vi "ABR-Plot Waveforms.vi"(0 "Array":dbl[][](array[numeric]), 2 "graph ref":refnum<vi>, 5 "dt (us)":dbl, 7 "Normalize traces":bool, 9 "Seqvals":dbl[](array[numeric]), 11 "error in (no error)":errorcluster, 12 "InnerVals":dbl[](array[numeric]), 13 "Threshold":dbl=nan) -> (15 "error out":errorcluster)   [LabVIEW 2020]
uses:
  epl-vi-lib/Utility VIs/Math VIs/LinSpace (x0-dx-npts).vi
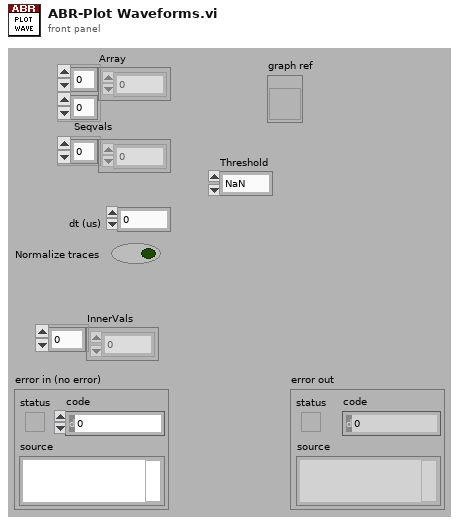
[diagram p1: front panel]
types:
  T1 = cluster{"Name":string, "Color":u32, "Style":u8, "Point Style":u8, "Name Visible":bool, "Allow Drag":bool, "Annotation Mode":u32, "Plot":i32, "Index":i32, "Position":cluster{"X":dbl, "Y":dbl}, "X Scale":u32, "Y Scale":u32, "Show Arrow":bool, "Lock Name":bool, "Plot Area":i32, "Label Offset":cluster{"X":dbl, "Y":dbl}}
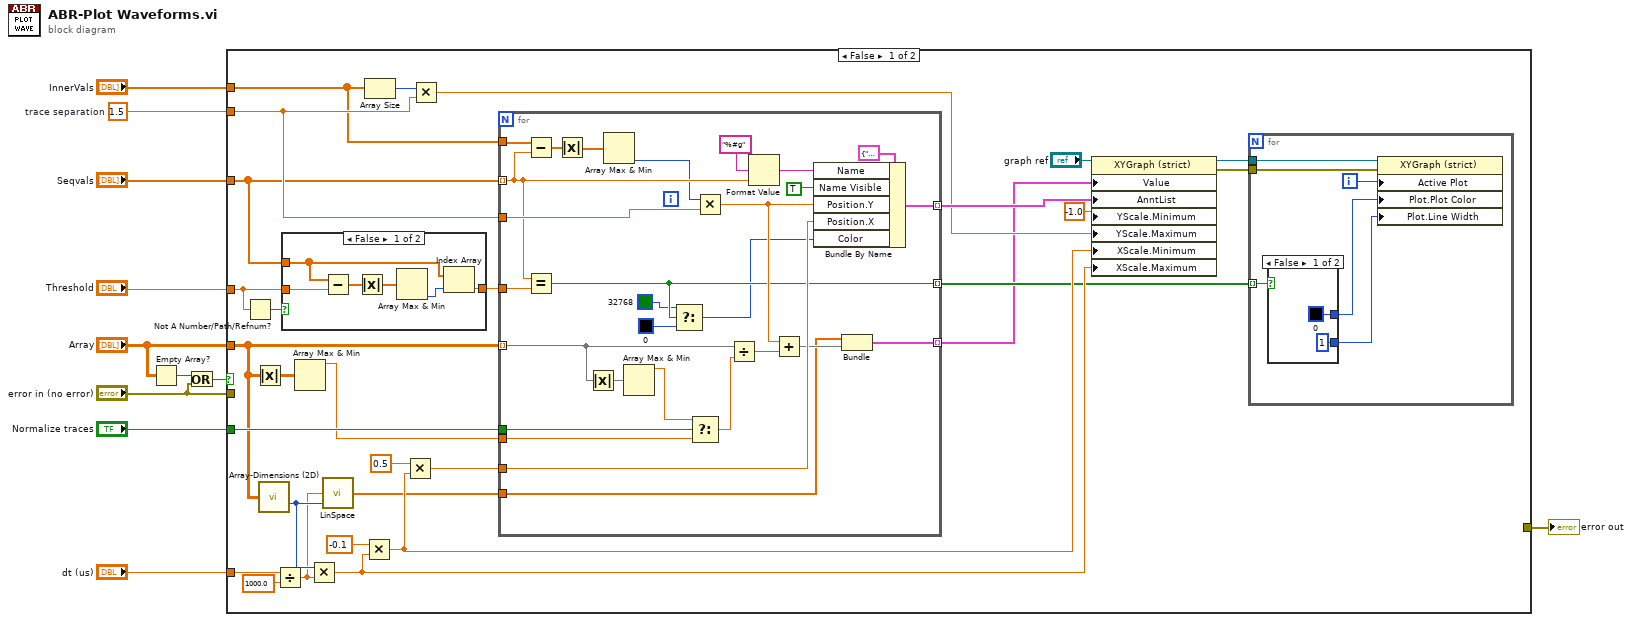
[diagram p0: block diagram]
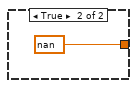
[diagram p2: hidden frame]
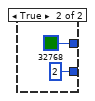
[diagram p3: hidden frame]
diagram:
  w8 = 1.5  # trace separation
  n1 = Empty Array?(array="Array") -> (empty?=w5:bool)
  n2 = Or(x=w5, y="error in (no error)") -> (x .or. y?=w3:bool)
  n3 = case shown="False" w3 {
    tunnel: "Array" -> [w30 _]
    tunnel: "dt (us)" -> [w40 _]
    tunnel: [_ w86] -> w10
    tunnel: "Seqvals" -> [w17 _]
    tunnel: w8 -> [w35 _]
    tunnel: "Normalize traces" -> [w33 _]
    tunnel: "InnerVals" -> [w24 _]
    tunnel: "error in (no error)" -> [_ w86]
    tunnel: "Threshold" -> [w14 _]
    frame False {
      n4 = Not A Number/Path/Refnum?(number/path/refnum=w14) -> (NaN/Path/Refnum?=w13:bool)
      n5 = Absolute Value(x=w30) -> (abs(x)=w32:dbl[][])
      n6 = call "Array-Dimensions (2D).vi"("2D Array"=w30) -> ("# columns"=w22:i32)  [unwired: 13 in, 1 out]
      n7 = Divide(x=w40, y=1000.0) -> (x/y=w20:dbl)
      n8 = case shown="False" w13 {
        tunnel: w17 -> [w43 _]
        tunnel: [w41 nan] -> w16
        tunnel: w14 -> [w44 _]
        frame False {
          n9 = Subtract(x=w43, y=w44) -> (x-y=w46:dbl[])
          n10 = Absolute Value(x=w46) -> (abs(x)=w45:dbl[])
          n11 = Array Max & Min(array=w45) -> (min index (indices)=w42:i32)  [unwired: 3 out]
          n12 = Index Array(array=w43, index=w42) -> (element=w41:dbl)
        }
        frame True {
        }
      }
      n13 = Array Max & Min(array=w32) -> (max value=w31:dbl)  [unwired: 3 out]
      n14 = Multiply(x=w22, y=w20) -> (x*y=w29:dbl)
      n15 = call-poly "LinSpace.vi"("npts"=w22, "dx"=w20) -> ("Array"=w21:dbl[])  [unwired: 2 in, 1 out]
      n16 = Multiply(x=-0.1, y=w29) -> (x*y=w26:dbl)
      n17 = Array Size(array=w24) -> (size(s)=w25:i32)
      n18 = Multiply(x=0.5, y=w26) -> (x*y=w23:dbl)
      n19 = Multiply(x=w25, y=w35) -> (x*y=w34:dbl)
      n20 = for {
        tunnel: w30 -> [w84] mode=indexing
        tunnel: [w69] -> w12 mode=indexing
        tunnel: w17 -> [w61] mode=indexing
        tunnel: [w80] -> w37 mode=indexing
        tunnel: w35 -> [w79]
        tunnel: w33 -> [w76]
        tunnel: w31 -> [w73]
        tunnel: w24 -> [w62]
        tunnel: w23 -> [w71]
        tunnel: w21 -> [w68]
        tunnel: w16 -> [w67]
        tunnel: [w66] -> w15 mode=indexing
        n21 = Subtract(x=w62, y=w61) -> (x-y=w60:dbl[])
        n22 = Equal?(x=w61, y=w67) -> (x = y?=w66:bool)
        n23 = Absolute Value(x=w60) -> (abs(x)=w59:dbl[])
        n24 = Absolute Value(x=w84) -> (abs(x)=w85:dbl[])
        n25 = Array Max & Min(array=w59) -> (min index (indices)=w58:i32)  [unwired: 3 out]
        n26 = Array Max & Min(array=w85) -> (max value=w75:dbl)  [unwired: 3 out]
        n27 = Select(t=u32 32768, s=w66, f=u32 0) -> (s? t:f=w63:u32)
        n28 = Select(t=w75, s=w76, f=w73) -> (s? t:f=w74:dbl)
        n29 = Multiply(x=w58, y=w79) -> (x*y=w78:dbl)
        n30 = Divide(x=w84, y=w74) -> (x/y=w77:dbl[])
        n31 = Format Value(format string="%#g", value (0)=w61) -> (output string=w81:string)  [unwired: 1 in]
        n32 = Add(x=w78, y=w77) -> (x+y=w70:dbl[])
        n33 = Bundle By Name(cluster=T1 {"Name"="", "Color"=0, "Style"=0, "Point Style"=0, "Name Visible"=FALSE, "Allow Drag"=FALSE, "Annotation Mode"=0, "Plot"=0, "Index"=0, "Position"={"X"=0.0, "Y"=0.0}, "X Scale"=0, "Y Scale"=0, "Show Arrow"=FALSE, "Lock Name"=FALSE, "Plot Area"=0, "Label Offset"={"X"=0.0, "Y"=0.0}} ("dummy annotation cluster\n(so we can bundle by name)"), "Name"=w81, "Name Visible"=TRUE, "Position.Y"=w78, "Position.X"=w71, "Color"=w63) -> (w80:T1)
        n34 = Bundle("Array"=w68, w70) -> (w69:cluster{"Array":dbl[], dbl[]})  [unwired: 1 in]
      }
      n35 = property class="XYGraph (strict)"(reference="graph ref", "Value"=w12, "AnntList"=w37, "YScale.Minimum"=-1.0 ("Y Scale.Range:Minimum"), "YScale.Maximum"=w34, "XScale.Minimum"=w26, "XScale.Maximum"=w29) -> (reference out=w19:refnum<vi>, error out=w18:errorcluster)  [unwired: 1 in]
      n36 = for {
        tunnel: w19 -> [w53]
        tunnel: w18 -> [w52]
        tunnel: w15 -> [w48] mode=indexing
        i -> [w51]
        n37 = case shown="False" w48 {
          tunnel: [u32 0 u32 32768] -> w50
          tunnel: [1 2] -> w49
          frame False {
          }
          frame True {
          }
        }
        n38 = property class="XYGraph (strict)"(reference=w53, error in=w52, "Active Plot"=w51, "Plot.Plot Color"=w50, "Plot.Line Width"=w49) -> ()  [unwired: 2 out]
      }
    }
    frame True {
    }
  }
  "error out" <- w10
